vi "LabView360-8.vi"() -> ()   [LabVIEW 2018]
panel:
  in  "数值 3":dbl
  in  "数值 2":dbl
  in  "布尔 2":bool
  in  "布尔":bool
  in  "Stop":bool
  in  "数值":dbl
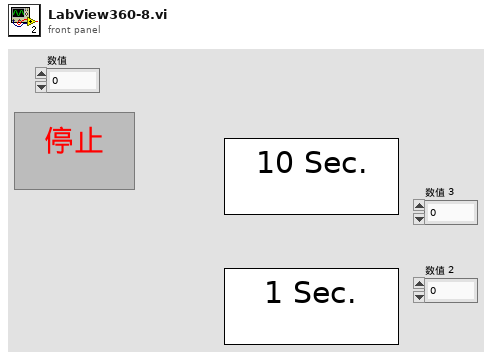
[diagram p1: front panel]
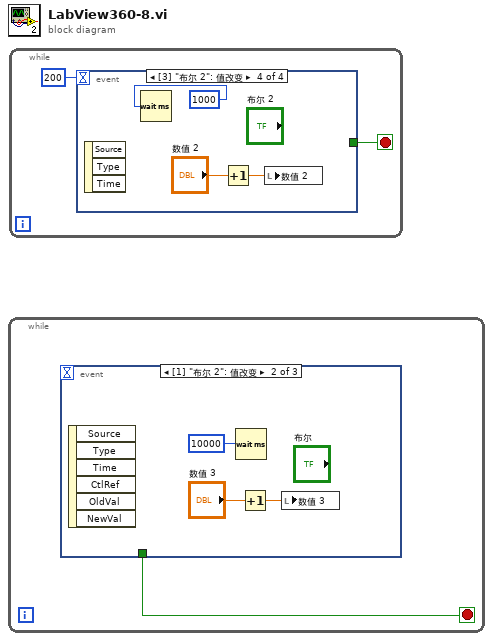
[diagram p0: block diagram]
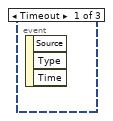
[diagram p2: hidden frame]
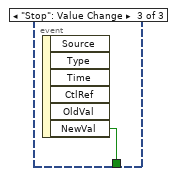
[diagram p3: hidden frame]
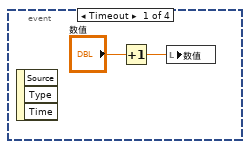
[diagram p4: hidden frame]
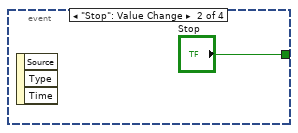
[diagram p5: hidden frame]
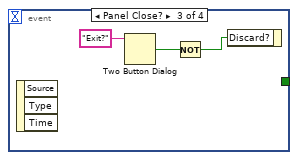
[diagram p6: hidden frame]
diagram:
  n1 = while {
    stop <- w1 stop-if-true
    n2 = event shown="[1] \"布尔 2\": 值改变" {
      selector: _ -> [_ _ _]
      dyn-events: _ -> [_ _ _]
      timeout: _ -> [_ _ _]
      tunnel: [_ _ w5] -> w1
      event Timeout {
        n3 = event-data() -> ()  [unwired: 1 in, 3 out]
      }
      event "布尔 2": Value Change {
        n4 = event-data() -> ()  [unwired: 1 in, 6 out]
        n5 = Wait (ms)(milliseconds to wait=u32 10000 ("等待时间（毫秒）")) -> ()  [unwired: 1 out]
        n6 = Increment(x="数值 3") -> (x+1=w3:dbl)
        n7 = local write "数值 3"(w3) -> ()
      }
      event "Stop": Value Change {
        n8 = event-data() -> ("NewVal"=w5:bool)  [unwired: 1 in, 5 out]
      }
    }
  }
  n9 = while {
    stop <- w7 stop-if-true
    n10 = event shown="[3] \"布尔 2\": 值改变" {
      selector: _ -> [_ _ _ _]
      dyn-events: _ -> [_ _ _ _]
      timeout: 200 -> [_ _ _ _]
      tunnel: [_ "Stop" _ _] -> w7
      event Timeout {
        n11 = event-data() -> ()  [unwired: 1 in, 3 out]
        n12 = Increment(x="数值") -> (x+1=w8:dbl)
        n13 = local write "数值"(w8) -> ()
      }
      event "Stop": Value Change {
        n14 = event-data() -> ()  [unwired: 1 in, 3 out]
      }
      event Panel Close? {
        n15 = event-data() -> ()  [unwired: 1 in, 3 out]
        n16 = Two Button Dialog(message="Exit?" ("消息")) -> (T button?=w11:bool)  [unwired: 2 in]
        n17 = Not(x=w11) -> (.not. x?=w12:bool)
        n18 = event-data("Discard?"=w12) -> ()  [unwired: 1 in, 1 out]
      }
      event "布尔 2": Value Change {
        n19 = event-data() -> ()  [unwired: 1 in, 3 out]
        n20 = Wait (ms)(milliseconds to wait=u32 1000 ("等待时间（毫秒）")) -> ()  [unwired: 1 out]
        n21 = Increment(x="数值 2") -> (x+1=w14:dbl)
        n22 = local write "数值 2"(w14) -> ()
      }
    }
  }
